vi "sweep table staff.vi"(7 "action":T1(ring), 9 "Sweep Table":dbl[][](array[numeric])=[[10.0, 400.0, 30.0], [220.0, 400.0, 0.0], [180.0, 200.0, 0.0], [220.0, 200.0, 0.0], [295.0, 200.0, 0.0], [0.0, 0.0, 0.0], [0.0, 0.0, 0.0], [0.0, 0.0, 0.0], [0.0, 0.0, 0.0], [0.0, 0.0, 0.0], [0.0, 0.0, 0.0], [0.0, 0.0, 0.0], [0.0, 0.0, 0.0], [0.0, 0.0, 0.0], [0.0, 0.0, 0.0], [295.0, 0.0, 0.0]], 10 "Sweep Rates , min/K IN":dbl[](array[numeric]), 11 "set temperature IN":dbl=300.0) -> (0 "date string Array":string[](array[string]), 1 "Sweep Table":dbl[][](array[numeric])=[[10.0, 400.0, 30.0], [220.0, 400.0, 0.0], [180.0, 200.0, 0.0], [220.0, 200.0, 0.0], [295.0, 200.0, 0.0], [0.0, 0.0, 0.0], [0.0, 0.0, 0.0], [0.0, 0.0, 0.0], [0.0, 0.0, 0.0], [0.0, 0.0, 0.0], [0.0, 0.0, 0.0], [0.0, 0.0, 0.0], [0.0, 0.0, 0.0], [0.0, 0.0, 0.0], [0.0, 0.0, 0.0], [295.0, 0.0, 0.0]], 2 "Sweep Rates , min/K":dbl[](array[numeric]), 3 "set temperature out":dbl=300.0)   [LabVIEW 2015]
uses:
  ITC Panel.ctl
  gas flow control.ctl
panel:
  out "Sweep Rates ,K/min":dbl[](array[numeric])
  in  "RUS loop":bool
  in  "gas flow control":T2={"ramp DOWN time step (sec)"=180, "DOWN step (%)"=1.0, "last check (min)"=0, "heater below"=TRUE, "heater above"=FALSE, "check every # min"=5.0, "upper"=12.0, "lower"=5.0, "heater"=2.965356705620467, "heater in range"=FALSE, "(total # of ramp DOWN steps)"=10, "ramp step (%)"=0.1, "DOWN time (min)"=30.0, "UP time (min)"=30.0, "(total # of ramp UP steps)"=10, "UP step (%)"=1.0, "ramp UP time step (sec)"=180, "set gas"=FALSE, "to"=3.8, "ramp UP"=TRUE, "ramp DOWN"=FALSE, "ramp UP steps so far"=1, "ramp UP in progress"=FALSE, "ramp DOWN steps so far "=0, "ramp DOWN in progress"=FALSE, "idle"=FALSE, "Gas flow, %"=90.0, "Control Gas"=FALSE, "state"=enum."ramp down"} {"Gas flow, %" format="%.2f"; "heater" format="%.2f"}
  in  "ITC panel":T3={"Locked"=FALSE, "Unlocked"=TRUE, "Remote"=FALSE, "Local"=TRUE, "in sweep"=TRUE, "start/stop sweep"=TRUE, "Sweep indicator"="IN sweep   1", "heater MANUAL"=FALSE, "heater AUTO"=TRUE, "ITC state"="X0A1C2S01H1L0\r", "gas MANUAL"=TRUE, "gas AUTO"=FALSE, "heater"=1.3, "gas flow %"=3.8} {"gas flow %" format="%.3g"; "heater" format="%.3g"}
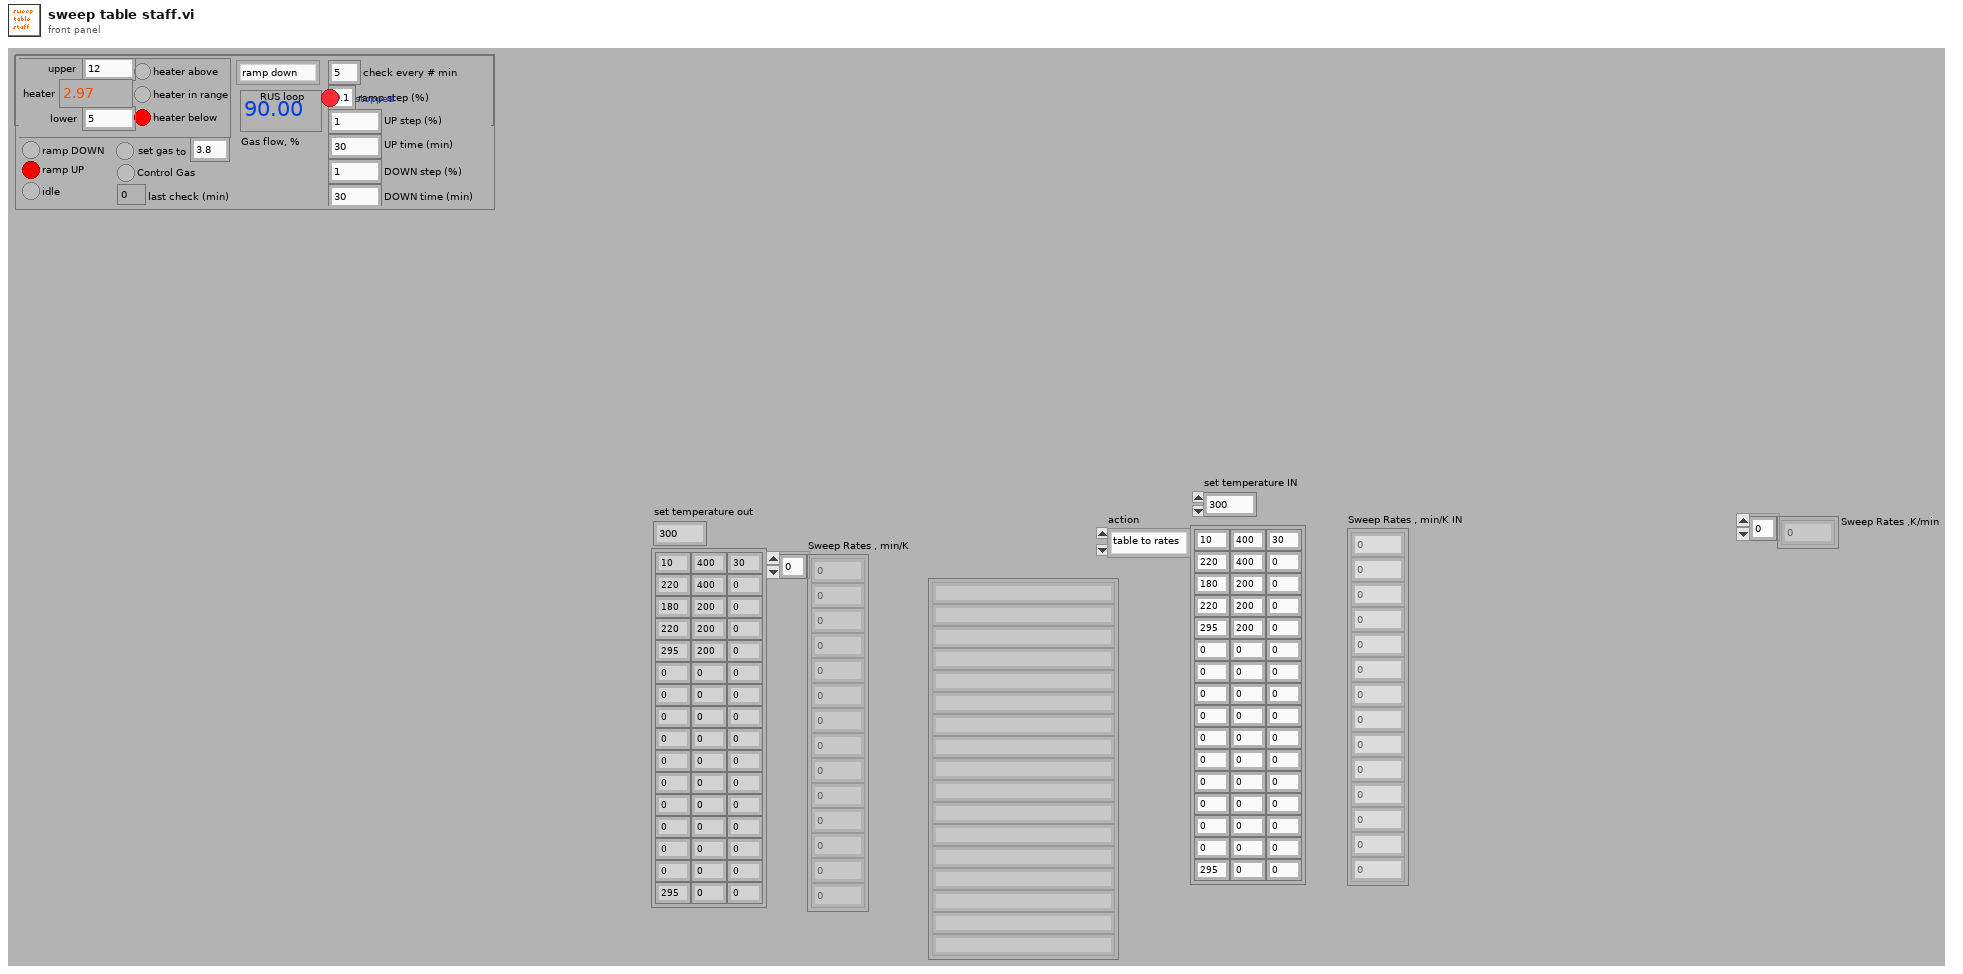
[diagram p1: front panel]
types:
  T1 = enum16{"table to rates", "rates to table", "other"}
  T2 = typedef "gas flow control.ctl" = cluster{"ramp DOWN time step (sec)":i32, "DOWN step (%)":dbl, "last check (min)":i32, "heater below":bool, "heater above":bool, "check every # min":dbl, "upper":dbl, "lower":dbl, "heater":dbl, "heater in range":bool, "(total # of ramp DOWN steps)":i32, "ramp step (%)":dbl, "DOWN time (min)":dbl, "UP time (min)":dbl, "(total # of ramp UP steps)":i32, "UP step (%)":dbl, "ramp UP time step (sec)":i32, "set gas":bool, "to":dbl, "ramp UP":bool, "ramp DOWN":bool, "ramp UP steps so far":i32, "ramp UP in progress":bool, "ramp DOWN steps so far ":i32, "ramp DOWN in progress":bool, "idle":bool, "Gas flow, %":dbl, "Control Gas":bool, "state":enum16{"normal", "ramp up", "ramp down"}}
  T3 = typedef "ITC Panel.ctl" = cluster{"Locked":bool, "Unlocked":bool, "Remote":bool, "Local":bool, "in sweep":bool, "start/stop sweep":bool, "Sweep indicator":string, "heater MANUAL":bool, "heater AUTO":bool, "ITC state":string, "gas MANUAL":bool, "gas AUTO":bool, "heater":dbl, "gas flow %":dbl}
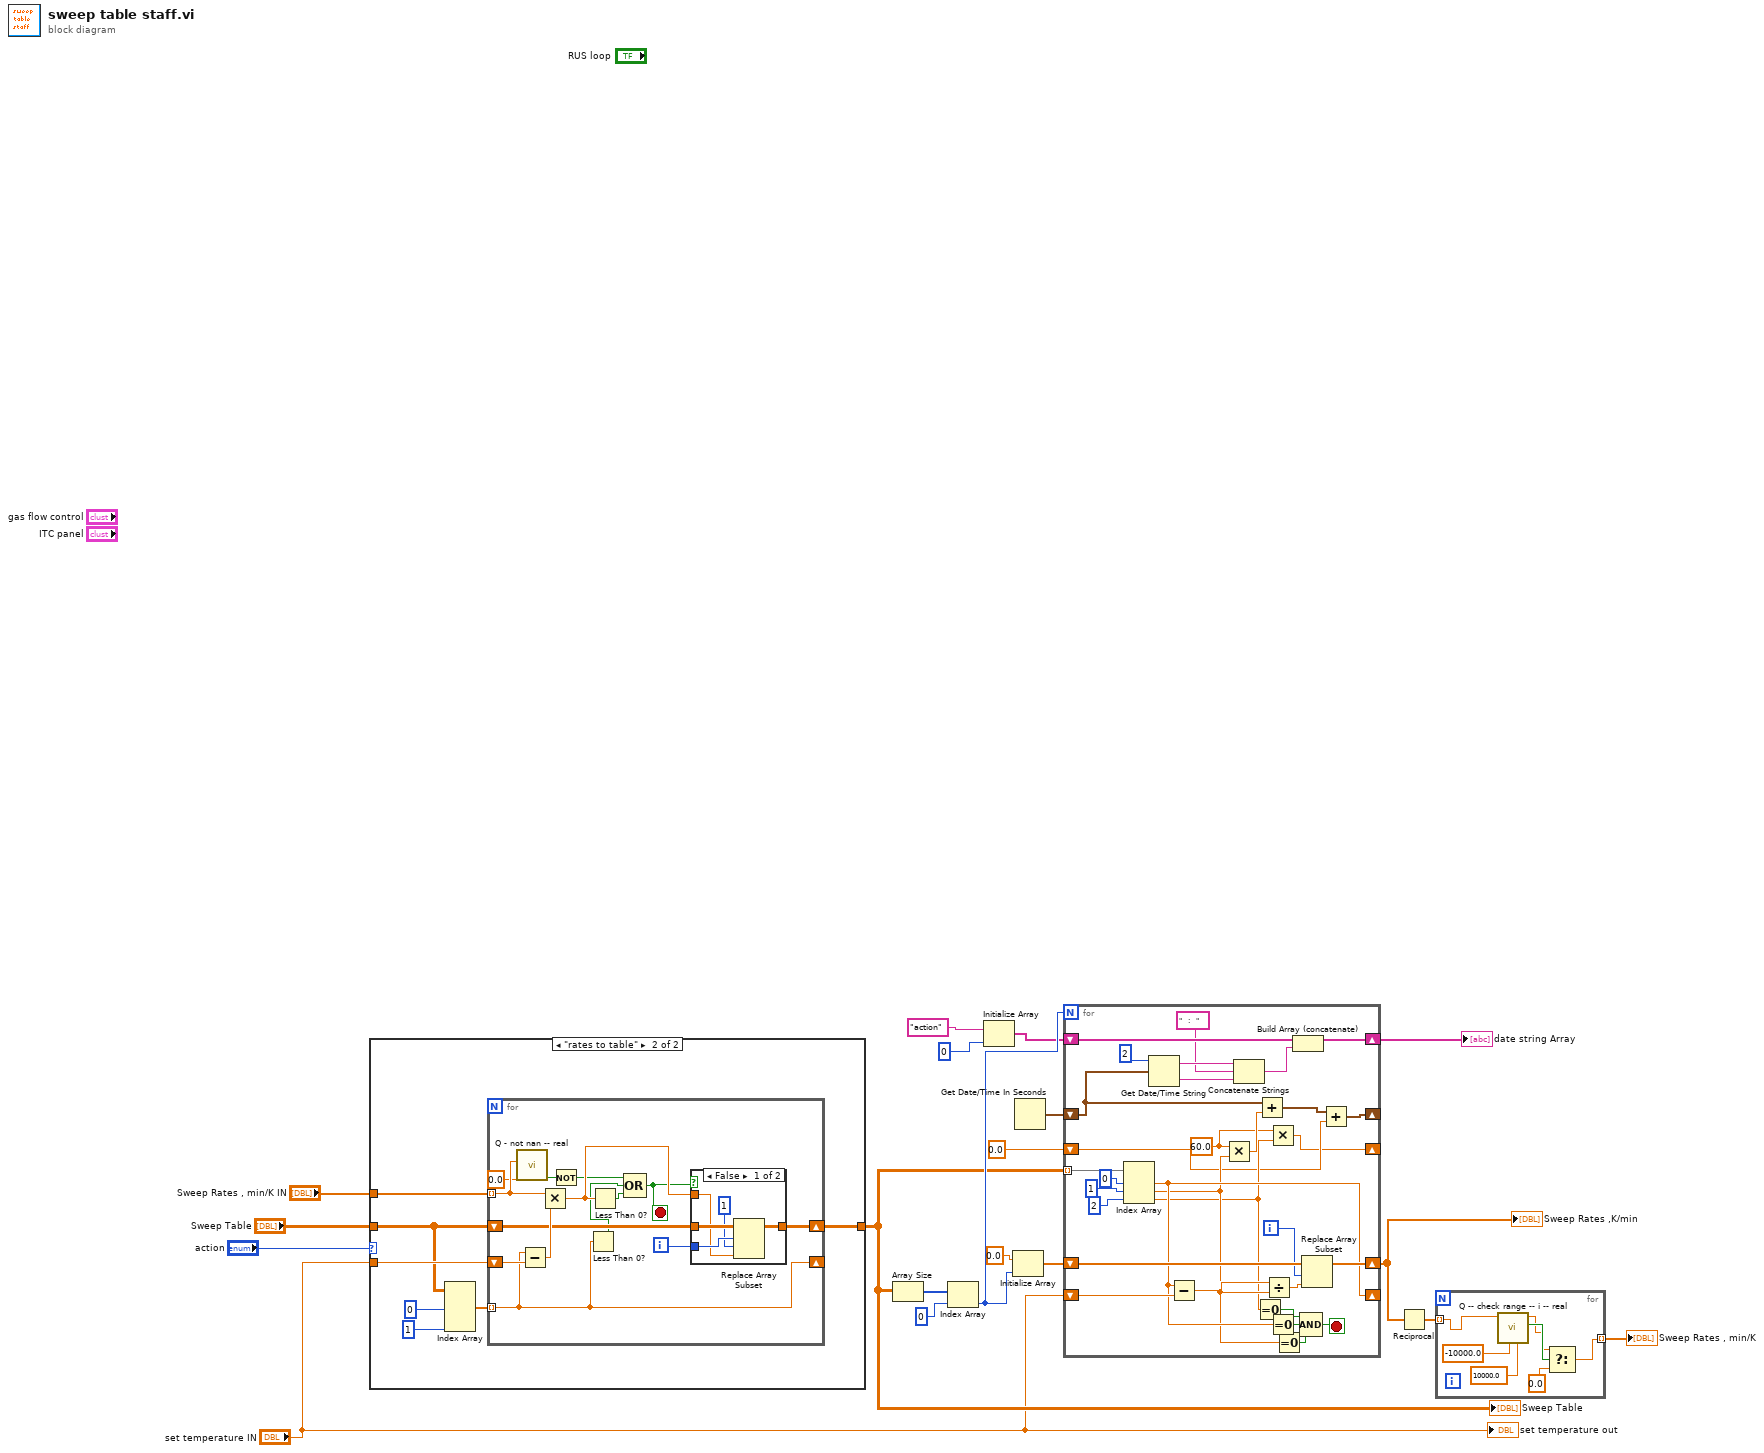
[diagram p0: block diagram]
diagram:
  n1 = case shown="\"rates to table\"" "action" {
    tunnel: "Sweep Table" -> [w20 w21]
    tunnel: [w20 w22] -> w4
    tunnel: "set temperature IN" -> [_ w27]
    tunnel: "Sweep Rates , min/K IN" -> [_ w25]
    frame "table to rates", Default {
    }
    frame "rates to table" {
      n2 = Index Array(array=w21, index (col) #1=0 ("index"), index (col) #2=1 ("index")) -> (element #1=w23:dbl[])  [unwired: 2 in, 1 out]
      n3 = for {
        shift-right: [w36] -> _
        shift-left: w27 -> [w41]
        tunnel: w23 -> [w36] mode=indexing
        tunnel: w25 -> [w29] mode=indexing
        shift-right: [w37] -> w22
        shift-left: w21 -> [w39]
        i -> [w38]
        stop <- w32 stop-if-true
        n4 = call "Q - not nan -- real.vi"("default"=0.0, "Numeric"=w29) -> ("Boolean"=w31:bool)  [unwired: 8 in, 1 out]
        n5 = Subtract(x=w36, y=w41) -> (x-y=w40:dbl)
        n6 = Multiply(x=w29, y=w40) -> (x*y=w35:dbl)
        n7 = Not(x=w31) -> (.not. x?=w30:bool)
        n8 = Less Than 0?(x=w36) -> (x < 0?=w33:bool)
        n9 = Less Than 0?(x=w35) -> (x < 0?=w34:bool)
        n10 = Compound Arithmetic op=OR(w30, w33, w34) -> (w32:bool)
        n11 = case shown="False" w32 {
          tunnel: w39 -> [w46 w47]
          tunnel: w38 -> [w45 _]
          tunnel: [w43 w47] -> w37
          tunnel: w35 -> [w42 _]
          frame False {
            n12 = Replace Array Subset(array=w46, new element=w42, index (row)=w45, index (col)=1 ("index")) -> (w43:dbl[][])
          }
          frame True {
          }
        }
      }
    }
  }
  "Sweep Table" <- w4
  n13 = Array Size(array=w4) -> (size(s)=w19:i32[])
  n14 = Index Array(array=w19, index=0) -> (element=w15:i32)
  n15 = Initialize Array("action" ("action"), 0 ("Sensor #")) -> (w11:string[])
  n16 = Initialize Array(0.0 ("element"), w15) -> (w16:dbl[])
  n17 = Get Date/Time In Seconds() -> (seconds since 1Jan1904=w14:timestamp)
  n18 = for {
    N: w15 -> [_]
    shift-right: [w75] -> w8
    shift-left: w16 -> [w77]
    tunnel: w4 -> [w74] mode=indexing
    shift-right: [w61] -> _
    shift-left: "set temperature IN" -> [w71]
    shift-right: [w55] -> _
    shift-left: w14 -> [w67]
    shift-right: [w68] -> w10
    shift-left: w11 -> [w69]
    shift-right: [w48] -> _
    shift-left: 0.0 ("element") -> [w49]
    i -> [w76]
    stop <- w50 stop-if-true
    w57 = 60.0 ("x")
    n19 = Index Array(array=w74, index #1=0 ("index"), index #2=1 ("index"), index #3=2 ("index")) -> (element #1=w61:dbl, element #2=w58:dbl, element #3=w54:dbl)
    n20 = Get Date/Time String(date format (0)=2 ("index"), seconds (now)=w67) -> (date string=w66:string, time string=w65:string)  [unwired: 1 in]
    n21 = Subtract(x=w61, y=w71) -> (x-y=w73:dbl)
    n22 = Multiply(x=w57, y=w58) -> (x*y=w70:dbl)
    n23 = Concatenate Strings(w66, "   :   " ("action"), w65) -> (w63:string)
    n24 = Equal To 0?(x=w54) -> (x = 0?=w51:bool)
    n25 = Add(x=w67, y=w70) -> (x+y=w56:timestamp)
    n26 = Divide(x=w73, y=w58) -> (x/y=w72:dbl)
    n27 = Multiply(x=w57, y=w54) -> (x*y=w48:dbl)
    n28 = Equal To 0?(x=w61) -> (x = 0?=w52:bool)
    n29 = Equal To 0?(x=w58) -> (x = 0?=w53:bool)
    n30 = Build Array (concatenate)(w69, w63) -> (w68:string[])
    n31 = Compound Arithmetic op=AND(w51, w52, w53) -> (w50:bool)
    n32 = Replace Array Subset(array=w77, new element=w72, index=w76) -> (w75:dbl[])
    n33 = Add(x=w56, y=w49) -> (x+y=w55:timestamp)
  }
  "date string Array" <- w10
  "Sweep Rates ,K/min" <- w8
  n34 = Reciprocal(x=w8) -> (1/x=w7:dbl[])
  n35 = for {
    tunnel: w7 -> [w85] mode=indexing
    tunnel: [w81] -> w6 mode=indexing
    n36 = call "Q -- check range -- i -- real.vi"("upper"=10000.0 ("element"), "lower"=-10000.0 ("element"), "number"=w85) -> ("in range?"=w83:bool, "number in range"=w82:dbl)  [unwired: 6 in, 1 out]
    n37 = Select(t=w82, s=w83, f=0.0 ("element")) -> (s? t:f=w81:dbl)
  }
  "Sweep Rates , min/K" <- w6
  "set temperature out" <- "set temperature IN"
